vi "Handle AREF XY COLROW.vi"(8 "error in":errorcluster, 11 "Referential in":refnum<class "Referential.lvclass">) -> (0 "error out":errorcluster, 2 "XY Vectors":cluster{"XY Matrix":T1}[](array[cluster]), 3 "Referential out":refnum<class "Referential.lvclass">)   [LabVIEW 2019, in "Referential.lvclass"]
uses:
  Referential.lvclass
  <vilib>/Analysis/Matrix/Datatypes/RealMatrix.ctl
  <vilib>/Analysis/baseanly.llb/Real A x B.vi
  <vilib>/Analysis/NI_AALBase.lvlib
  <vilib>/Analysis/Matrix/NI_Matrix.lvlib
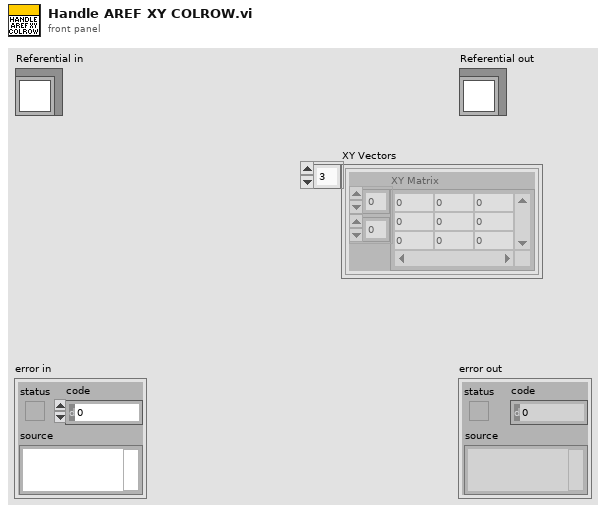
[diagram p1: front panel]
types:
  T1 = typedef "NI_Matrix.lvlib/RealMatrix.ctl" = dbl[][]
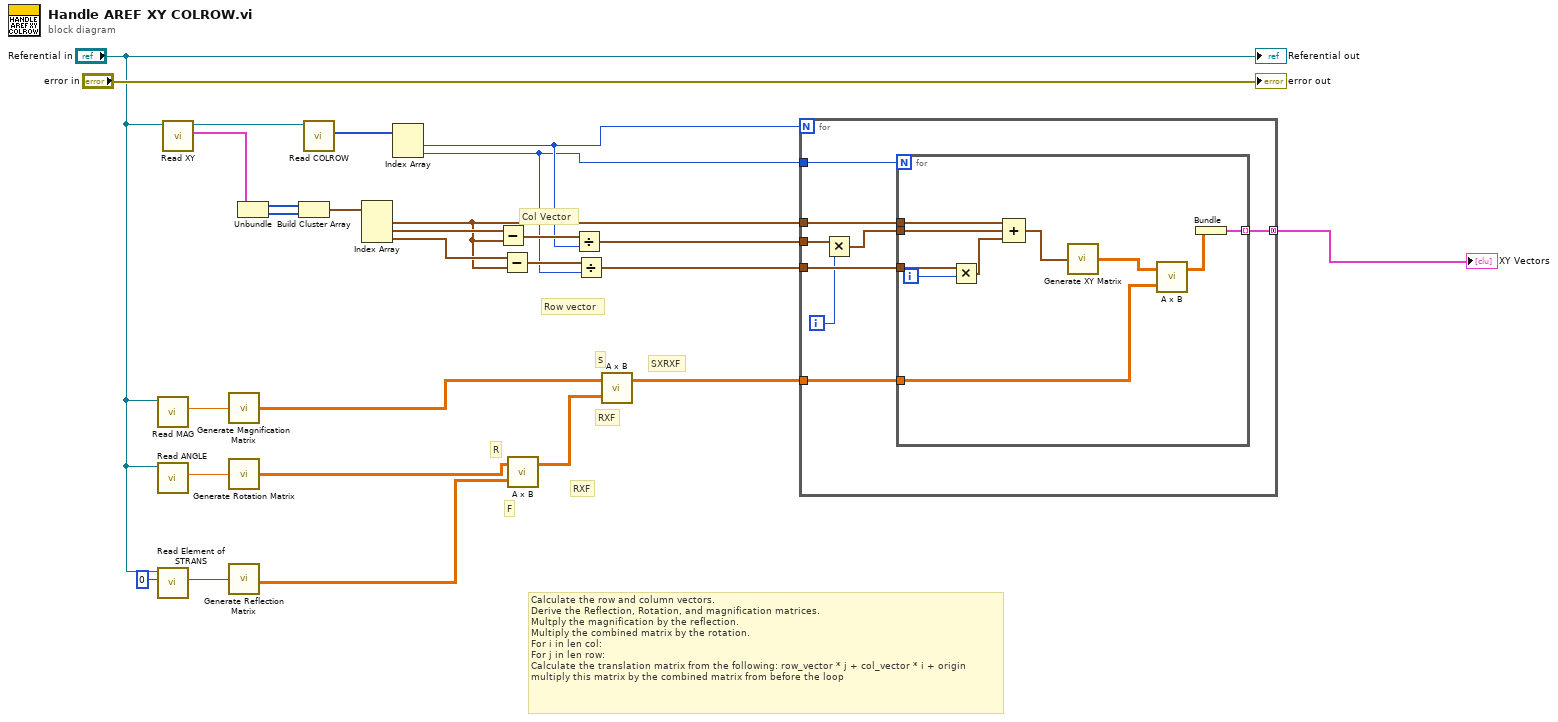
[diagram p0: block diagram]
diagram:
  # "SXRXF"
  # "RXF"
  # "S"
  # "RXF"
  # "R"
  # "F"
  # "Calculate the row and column vectors.\nDerive the Reflection, Rotation, and magnification matrices. \nMultply the magnification by the reflection.\nMultiply the combined matrix by the rotation.\nFor i in len col:\nFor j in len row:\nCalculate the translation matrix from the following: row_vector * j + col_vector * i + origin\nmultiply this matrix by the combined matrix from before the loop"
  # "Row vector"
  # "Col Vector"
  n1 = call-dynamic "Read MAG.vi"("Referential in"="Referential in") -> ("MAG"=w11:dbl)  [unwired: 8 in, 2 out]
  n2 = call-dynamic "Read ANGLE.vi"("Referential in"="Referential in") -> ("ANGLE"=w12:dbl)  [unwired: 8 in, 2 out]
  n3 = call-dynamic "Read Element of STRANS.vi"("index"=0, "Referential in"="Referential in") -> ("Bit"=w2:bool)  [unwired: 7 in, 2 out]
  n4 = call-dynamic "Read XY.vi"("Element in"="Referential in") -> ("XY"=w24:cluster{"X":i32[], "Y":i32[]}, "Element out"=w23:refnum<class "Referential.lvclass">)  [unwired: 8 in, 1 out]
  n5 = call "Generate Magnification Matrix.vi"("Magnification"=w11) -> ("Magnification Matrix"=w7:T1)
  n6 = call "Generate Rotation Matrix.vi"("Angle"=w12) -> ("Rotation Matrix"=w6:T1)
  n7 = call "Generate Reflection Matrix.vi"("Bit"=w2) -> ("Reflection Matrix"=w3:T1)
  n8 = Unbundle(w24) -> ("X"=w27:i32[], "Y"=w26:i32[])
  n9 = Build Cluster Array(w27, w26) -> (w25:cluster{"X":i32, "X":i32}[])
  n10 = call-dynamic "Read COLROW.vi"("Referential in"=w23) -> ("COLROW"=w22:i16[])  [unwired: 8 in, 2 out]
  n11 = Index Array(array=w25) -> (element #1=w10:cluster{"X":i32, "X":i32}, element #2=w21:cluster{"X":i32, "X":i32}, element #3=w20:cluster{"X":i32, "X":i32})  [unwired: 3 in]
  n12 = Index Array(array=w22) -> (element #1=w17:i16, element #2=w16:i16)  [unwired: 2 in]
  n13 = Subtract(x=w21, y=w10) -> (x-y=w19:cluster{"X":i32, "X":i32})
  n14 = Subtract(x=w20, y=w10) -> (x-y=w18:cluster{"X":i32, "X":i32})
  n15 = call-poly <vilib>:"A x B.vi"("B"=w3, "A"=w6) -> ("A x B"=w5:T1)  [unwired: 1 out]
  n16 = Divide(x=w19, y=w17) -> (x/y=w15:cluster{"X":dbl, "X":dbl})
  n17 = Divide(x=w18, y=w16) -> (x/y=w14:cluster{"X":dbl, "X":dbl})
  n18 = call-poly <vilib>:"A x B.vi"("B"=w5, "A"=w7) -> ("A x B"=w9:T1)  [unwired: 1 out]
  n19 = for {
    N: w17 -> [_]
    tunnel: w10 -> [w34]
    tunnel: w16 -> [w35]
    tunnel: w15 -> [w32]
    tunnel: w14 -> [w33]
    tunnel: [w29] -> w4 mode=concatenating
    tunnel: w9 -> [w28]
    i -> [w31]
    n20 = Multiply(x=w32, y=w31) -> (x*y=w30:cluster{"X":dbl, "X":dbl})
    n21 = for {
      N: w35 -> [_]
      tunnel: w34 -> [w39]
      tunnel: w33 -> [w44]
      tunnel: w30 -> [w43]
      tunnel: [w41] -> w29 mode=indexing
      tunnel: w28 -> [w37]
      i -> [w45]
      n22 = Multiply(x=w44, y=w45) -> (x*y=w42:cluster{"X":dbl, "X":dbl})
      n23 = Compound Arithmetic op=ADD(w39, w43, w42) -> (w40:cluster{"X":dbl, "X":dbl})
      n24 = call "Generate XY Matrix.vi"("XY"=w40) -> ("XY Matrix"=w38:T1)
      n25 = call-poly <vilib>:"A x B.vi"("B"=w37, "A"=w38) -> ("A x B"=w36:T1)  [unwired: 1 out]
      n26 = Bundle("A x B"=w36) -> (w41:cluster{"A x B":T1})  [unwired: 1 in]
    }
  }
  "XY Vectors" <- w4
  "error out" <- "error in"
  "Referential out" <- "Referential in"
